vi "Display and Log Process.vi"(10 "Parameters":variant, 11 "Process":refnum<class "Process.lvclass">) -> ()   [LabVIEW 2027, in "VS Inline Async API (Express).lvlib"]
uses:
  VS Inline Async API (Express).lvlib
  Process/Process.lvclass
  VS Inline Async API (Express)/Types/Error Handling Settings.ctl
  Process/Process.lvclass/Process.ctl
  <vilib>/Utility/error.llb/Trim Whitespace (string).vi
  Process/Data Member Access/Read Name.vi
  Process/Data Member Access/Read Process.Trigger.vi
  Process/Data Member Access/Read Process.Stop.vi
  SubVIs/Error.Message.Format.vi
  SubVIs/Error.Tags.Check.vi
  <vilib>/Utility/error.llb/Trim Whitespace One-Sided.vi
  <vilib>/Utility/error.llb/Error Code Database.vi
  <vilib>/Utility/error.llb/Find Tag.vi
  <vilib>/NI VeriStand/Custom Device Tools/Custom Device Utility Library/Custom Device Utility Library.lvlib
  VS Inline Async API (Express)/VS Inline Async API (Express).lvclass
  <vilib>/Utility/SystemLogging/NI_SystemLogging.lvlib
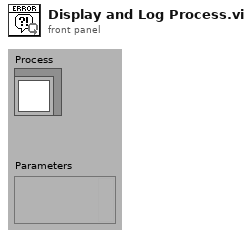
[diagram p1: front panel]
types:
  T1 = typedef "VS Inline Async API (Express).lvlib/VS Inline Async API (Express).lvclass/Error Handling Settings.ctl" = cluster{"Write to SystemLog (F)":bool}
  T2 = cluster{"read mode":enum16{"polling", "blocking"}, "write mode":enum16{"polling", "blocking"}}
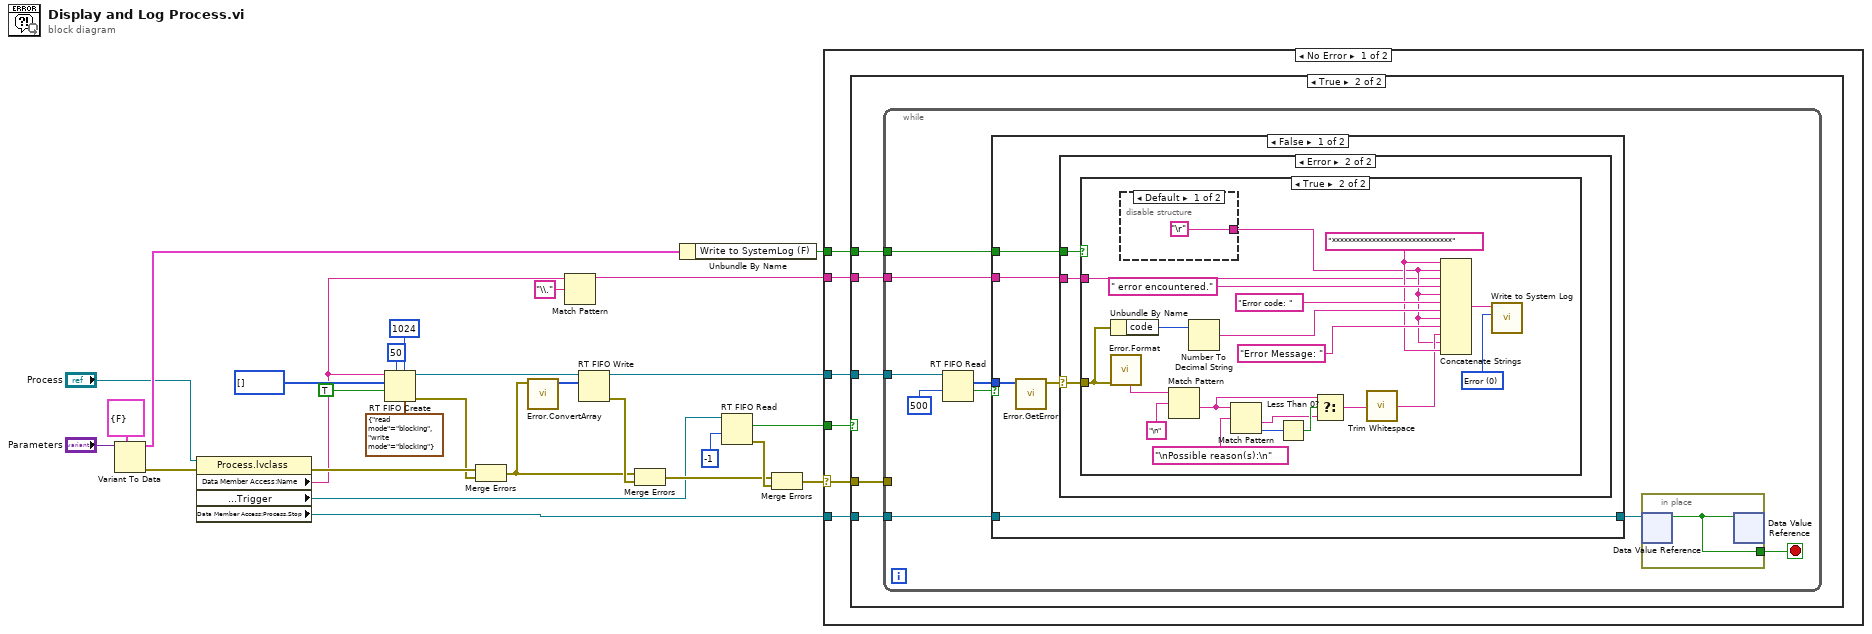
[diagram p0: block diagram]
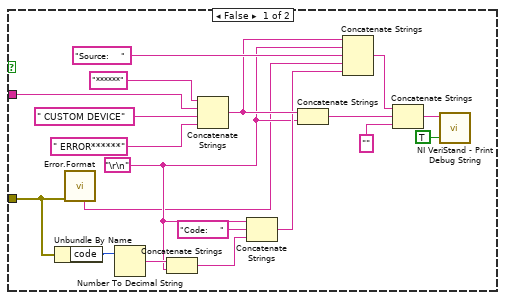
[diagram p4: hidden frame]
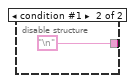
[diagram p5: hidden frame]
diagram:
  n1 = Variant To Data(type=T1 {"Write to SystemLog (F)"=FALSE}, Variant="Parameters") -> (data=w6:T1, error out=w9:errorcluster)  [unwired: 1 in]
  n2 = property class="Process.lvclass"(reference="Process", error in=w9) -> (error out=w26:errorcluster, "Data Member Access:Name"=w4:string, "Data Member Access:Process.Trigger"=w12:refnum<k33>, "Data Member Access:Process.Stop"=w27:refnum<data-value>)  [unwired: 1 out]
  n3 = RT FIFO Create(0:w4, 1:u8[] [], 2:TRUE ("create if not found? (T)"), 4:u32 50 ("size (10)"), 6:u32 1024 ("elements in array (1)"), 7:T2 {"read mode"=enum."blocking", "write mode"=enum."blocking"} ("r/w modes (polling,polling)")) -> (8:w28:refnum<k33>, 11:w24:errorcluster)  [unwired: 2 in, 1 out]
  n4 = Merge Errors(w26, w24) -> (w23:errorcluster)
  n5 = call "Error.ConvertArray.vi"("error in"=w23) -> ("Msg"=w20:u8[])  [unwired: 10 in]
  n6 = Match Pattern(string=w4, regular expression="\\.") -> (before substring=w3:string)  [unwired: 1 in, 3 out]
  n7 = RT FIFO Write(0:w28, 1:w20) -> (8:w10:refnum<k33>, 11:w25:errorcluster)  [unwired: 3 in, 2 out]
  n8 = Merge Errors(w23, w25) -> (w14:errorcluster)
  n9 = Unbundle By Name(w6) -> ("Write to SystemLog (F)"=w5:bool)
  n10 = RT FIFO Read(0:w12, 2:-1 ("timeout in ms (-1)")) -> (9:w11:bool, 11:w15:errorcluster)  [unwired: 2 in, 3 out]
  n11 = Merge Errors(w14, w15) -> (w13:errorcluster)
  n12 = case shown="No Error" w13 {
    selector: w13 -> [w30 _]
    tunnel: w11 -> [w34 _]
    tunnel: w3 -> [w33 _]
    tunnel: w10 -> [w32 _]
    tunnel: w27 -> [w31 _]
    tunnel: w5 -> [w29 _]
    frame No Error {
      n13 = case shown="True" w34 {
        tunnel: w32 -> [_ w39]
        tunnel: w33 -> [_ w38]
        tunnel: w30 -> [_ w37]
        tunnel: w31 -> [_ w36]
        tunnel: w29 -> [_ w35]
        frame False {
        }
        frame True {
          n14 = while {
            tunnel: w39 -> [w48]
            tunnel: w38 -> [w47]
            tunnel: w37 -> [_]
            tunnel: w36 -> [w41]
            tunnel: w35 -> [w40]
            stop <- w43 stop-if-true
            n15 = RT FIFO Read(0:w48, 2:500 ("timeout in ms (-1)")) -> (9:w46:u8[], 10:w44:bool)  [unwired: 2 in, 3 out]
            n16 = case shown="False" w44 {
              tunnel: w46 -> [w53 _]
              tunnel: w47 -> [w52 _]
              tunnel: [w54 w99] -> w42
              tunnel: w41 -> [w54 w99]
              tunnel: w40 -> [w50 _]
              frame False {
                n17 = call "Error.GetError.vi"("Msg"=w53) -> ("error out"=w51:errorcluster)  [unwired: 10 in]
                n18 = case shown="Error" w51 {
                  selector: w51 -> [_ w56]
                  tunnel: w52 -> [_ w57]
                  tunnel: w50 -> [_ w55]
                  frame No Error {
                  }
                  frame Error {
                    n19 = case shown="True" w55 {
                      tunnel: w57 -> [w64 w80]
                      tunnel: w56 -> [w59 w78]
                      frame False {
                        w63 = "\r\n"
                        n20 = Unbundle By Name(w59) -> ("code"=w66:i32)
                        n21 = call "Error.Format.vi"("error in (no error)"=w59) -> ("message"=w58:string)  [unwired: 6 in, 4 out]
                        n22 = Number To Decimal String(number=w66) -> (decimal integer string=w74:string)  [unwired: 1 in]
                        n23 = Concatenate Strings(w74, w63) -> (w65:string)
                        n24 = Concatenate Strings("******" ("String"), w64, " CUSTOM DEVICE" ("String"), " ERROR******" ("String")) -> (w71:string)
                        n25 = Concatenate Strings(w63, "Code:    " ("String"), w65) -> (w70:string)
                        n26 = Concatenate Strings(w71, w63) -> (w68:string)
                        n27 = Concatenate Strings(w71, w63, "Source:    " ("String"), w58, w70) -> (w69:string)
                        n28 = Concatenate Strings(w69, w68, "" ("Message")) -> (w62:string)
                        n29 = call <vilib>:"NI VeriStand - Print Debug String.vi"("Add to log file? (F)"=TRUE ("Add to log file? (T)"), "Message"=w62) -> ()  [unwired: 9 in, 1 out]
                      }
                      frame True {
                        w91 = "******************************" ("string")
                        w96 = 0 items=["Error", "Warning", "Informational"] ("severity")
                        n30 = Unbundle By Name(w78) -> ("code"=w77:i32)
                        n31 = call "Error.Format.vi"("error in (no error)"=w78) -> ("message"=w79:string)  [unwired: 6 in, 4 out]
                        n32 = disable-structure shown="Default" {
                          disable-tunnel: ["\r" "\n"] -> w82
                          frame condition #0 (active) {
                          }
                          frame condition #1 {
                          }
                        }
                        n33 = Match Pattern(string=w79, regular expression="\n" ("string")) -> (after substring=w86:string)  [unwired: 1 in, 3 out]
                        n34 = Number To Decimal String(number=w77) -> (decimal integer string=w93:string)  [unwired: 1 in]
                        n35 = Match Pattern(string=w86, regular expression="\nPossible reason(s):\n" ("string")) -> (after substring=w85:string, offset past match=w88:i32)  [unwired: 1 in, 2 out]
                        n36 = Less Than 0?(x=w88) -> (x < 0?=w87:bool)
                        n37 = Select(t=w86, s=w87, f=w85) -> (s? t:f=w84:string)
                        n38 = call-poly <vilib>:"Trim Whitespace.vi"("string"=w84) -> ("trimmed string"=w83:string)  [unwired: 1 in]
                        n39 = Concatenate Strings(w91, w82, w80, " error encountered." ("String"), w82, "Error code: " ("string"), w93, w82, "Error Message: " ("string"), w83, w82, w91) -> (w81:string)
                        n40 = call <vilib>:"Write to System Log.vi"("severity"=w96, "message"=w81) -> ()  [unwired: 9 in, 1 out]
                      }
                    }
                  }
                }
              }
              frame True {
              }
            }
            n41 = in-place {
              in-place-border: [w49] -> w43
              n42 = in-place-dvr #1(w42) -> (w49:bool)  [unwired: 1 out]
              n43 = in-place-dvr #1(w49) -> ()  [unwired: 2 out]
            }
          }
        }
      }
    }
    frame Error {
    }
  }
